vi "Passive Active Measurement.vi"(0 "Sequence Context":refnum<k7>, 1 "test case":T2=enum."TC16", 2 "n rows":i32=21, 3 "Idle Offset Voltage":dbl format="%.6g", 4 "Pulse Characteristics":T1={"Pulses per Cycle"=4, "Load Resistance (Ohms)"=nan, "Krec Value"=2, "Recovery Mode (T=Active)"=TRUE, "Target Stim Currents (Amps)"=[]}, 5 "error in":errorcluster, 6 "step name":string="Sequence Step General: Name", 7 "Repetitions in the Waveform (4)":i32=4, 8 "filepath":path) -> (19 "error out":errorcluster)   [LabVIEW 2010]
uses:
  Active Output Test Cases.ctl
panel:
  # "Enter Target Current\nfor each in array below"
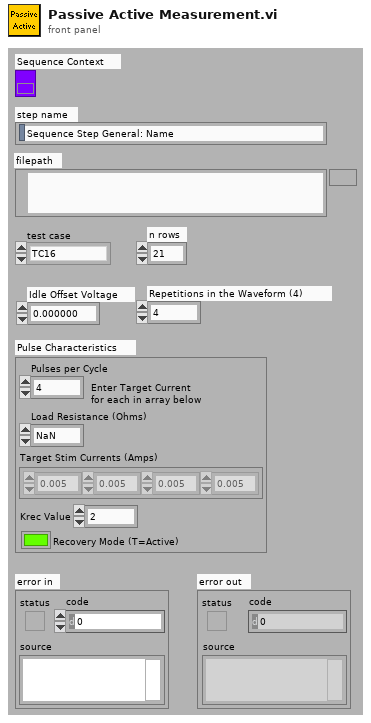
[diagram p1: front panel]
types:
  T1 = cluster{"Pulses per Cycle":i32, "Load Resistance (Ohms)":dbl, "Krec Value":i32, "Recovery Mode (T=Active)":bool, "Target Stim Currents (Amps)":dbl[]}
  T2 = typedef "Active Output Test Cases.ctl" = enum16{"TC1", "TC2", "TC3", "TC4", "TC5", "TC6", "TC7", "TC8", "TC9", "TC10", "TC11", "TC12", "TC13", "TC14", "TC15", "TC16", "TC17", "TC18", "TC19", "TC20", "TC21", "TC22", "TC23", "TC24", "TC25", "TC26", "TC27", "TC28", "TC29", "TC30", "TC31", "TC32", "TC33", "TC34", "TC35", "TC36"}
  T3 = typedef "Analyze Ouptut Parameters.ctl" = cluster{"Stim Amplitude":dbl[], "Stim Pulse Width":dbl[], "Interphase Delay":dbl[], "Recovery Amplitude":dbl[], "Recovery PW":dbl[], "Recovery Holdoff":dbl[], "Frequency":dbl, "Avg CBC Width":dbl, "Avg. CBC Holdoff":dbl, "Avg. CBC Amplitude":dbl}
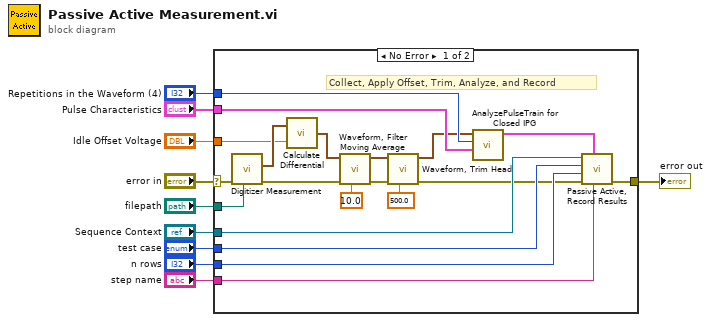
[diagram p0: block diagram]
diagram:
  n1 = case shown="No Error" "error in" {
    selector: "error in" -> [w21 w31]
    tunnel: "filepath" -> [w30 _]
    tunnel: "Idle Offset Voltage" -> [w28 _]
    tunnel: "Sequence Context" -> [w27 _]
    tunnel: "test case" -> [w26 _]
    tunnel: "n rows" -> [w25 _]
    tunnel: [w24 w31] -> w5
    tunnel: "step name" -> [w22 _]
    tunnel: "Pulse Characteristics" -> [w20 _]
    tunnel: "Repetitions in the Waveform (4)" -> [w19 _]
    frame No Error {
      # "Collect, Apply Offset, Trim, Analyze, and Record"
      n2 = call "Digitizer Measurement.vi"("filepath"=w30, "error in"=w21) -> ("error out"=w15:errorcluster, "waveform array"=w29:waveform(dbl)[])  [unwired: 8 in]
      n3 = call "Calculate Differential.vi"("Idle Offset Voltage"=w28, "Waveform Array In"=w29) -> ("Waveform Out"=w12:waveform(dbl))
      n4 = call "Waveform, Filter Moving Average.vi"("Average Size"=10.0, "error in"=w15, "waveform"=w12) -> ("error out"=w14:errorcluster, "waveform out"=w13:waveform(dbl))  [unwired: 5 in]
      n5 = call "Waveform, Trim Head.vi"("error in"=w14, "waveform"=w13, "interval (250 us)"=500.0) -> ("error out"=w18:errorcluster, "waveform out"=w17:waveform(dbl))  [unwired: 5 in, 1 out]
      n6 = call "AnalyzePulseTrain for Closed IPG.vi"("Pulse Characteristics"=w20, "Repetitions in the Input Waveform"=w19, "Waveform In"=w17) -> ("Waveform Parameters"=w23:T3)  [unwired: 6 in]
      n7 = call "Passive Active, Record Results.vi"("step name"=w22, "Waveform Parameters"=w23, "error in"=w18, "n rows"=w25, "test case"=w26, "Sequence Context"=w27) -> ("error out"=w24:errorcluster)  [unwired: 4 in, 1 out]
    }
    frame Error {
    }
  }
  "error out" <- w5
